vi "Update Connection Page Visibility.vi"(10 "Connection Type":T2, 11 "Config References":T1) -> (0 "error out":errorcluster)   [LabVIEW 2015, in "SystemLink editor node.lvclass"]
doc: "Update visible controls on \"Connection Configuration\" page of SystemLink Tag editor node."
uses:
  SystemLink editor node.lvclass
  module/configuration/Connection Type.ctl
  module/configuration/SystemLink configuration.lvclass
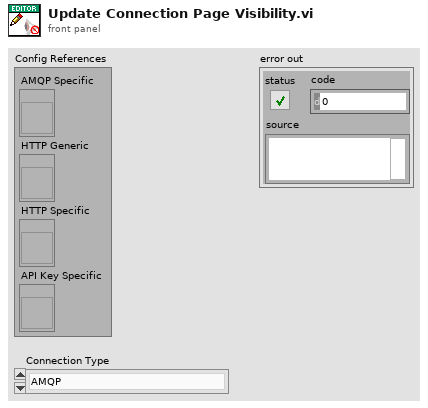
[diagram p1: front panel]
types:
  T1 = cluster{"AMQP Specific":refnum<vi>, "HTTP Generic":refnum<vi>, "HTTP Specific":refnum<vi>, "API Key Specific":refnum<vi>}
  T2 = typedef "SystemLink configuration.lvclass/Connection Type.ctl" = enum16{"AMQP", "HTTP", "API Key (SystemLink Cloud)"}
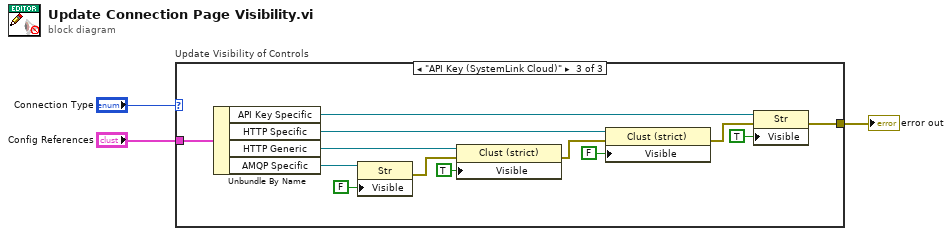
[diagram p0: block diagram]
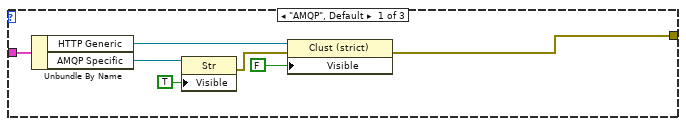
[diagram p2: hidden frame]
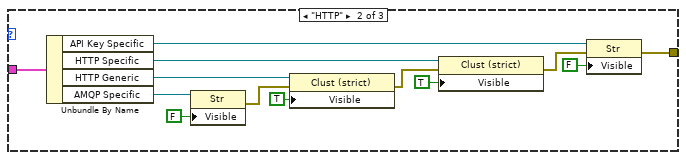
[diagram p3: hidden frame]
diagram:
  n1 = case "Update Visibility of Controls" shown="\"API Key (SystemLink Cloud)\"" "Connection Type" {
    tunnel: "Config References" -> [w10 w23 w36]
    tunnel: [w4 w11 w24] -> w1
    frame "AMQP", Default {
      n2 = Unbundle By Name(w10) -> ("HTTP Generic"=w7:refnum<vi>, "AMQP Specific"=w9:refnum<vi>)
      n3 = property class="Str"(reference=w9, "Visible"=TRUE) -> (error out=w6:errorcluster)  [unwired: 1 in, 1 out]
      n4 = property class="Clust (strict)"(reference=w7, error in=w6, "Visible"=FALSE) -> (error out=w4:errorcluster)  [unwired: 1 out]
    }
    frame "HTTP" {
      n5 = Unbundle By Name(w23) -> ("API Key Specific"=w13:refnum<vi>, "HTTP Specific"=w17:refnum<vi>, "HTTP Generic"=w20:refnum<vi>, "AMQP Specific"=w22:refnum<vi>)
      n6 = property class="Str"(reference=w22, "Visible"=FALSE) -> (error out=w18:errorcluster)  [unwired: 1 in, 1 out]
      n7 = property class="Clust (strict)"(reference=w20, error in=w18, "Visible"=TRUE) -> (error out=w16:errorcluster)  [unwired: 1 out]
      n8 = property class="Clust (strict)"(reference=w17, error in=w16, "Visible"=TRUE) -> (error out=w14:errorcluster)  [unwired: 1 out]
      n9 = property class="Str"(reference=w13, error in=w14, "Visible"=FALSE) -> (error out=w11:errorcluster)  [unwired: 1 out]
    }
    frame "API Key (SystemLink Cloud)" {
      n10 = Unbundle By Name(w36) -> ("API Key Specific"=w26:refnum<vi>, "HTTP Specific"=w30:refnum<vi>, "HTTP Generic"=w33:refnum<vi>, "AMQP Specific"=w35:refnum<vi>)
      n11 = property class="Str"(reference=w35, "Visible"=FALSE) -> (error out=w31:errorcluster)  [unwired: 1 in, 1 out]
      n12 = property class="Clust (strict)"(reference=w33, error in=w31, "Visible"=TRUE) -> (error out=w29:errorcluster)  [unwired: 1 out]
      n13 = property class="Clust (strict)"(reference=w30, error in=w29, "Visible"=FALSE) -> (error out=w27:errorcluster)  [unwired: 1 out]
      n14 = property class="Str"(reference=w26, error in=w27, "Visible"=TRUE) -> (error out=w24:errorcluster)  [unwired: 1 out]
    }
  }
  "error out" <- w1
